vi "ReadRootPath.vi"(1 "LibBuildRootFolderName":string="ECU_Diagnose") -> (15 "Root path":path)   [LabVIEW 2020, in "DAQ.lvlib" / "DAQ_Base.lvclass"]
uses:
  DAQ_Base.lvclass
panel:
  out "匹配后偏移量":i32
  out "匹配后偏移量":i32
  out "子字符串之前":string
  out "应用程序:类别":T1(ring)
  out "原本路径":path
  # "以builds命名，并且exe直接放在builds下就不需要填这个"
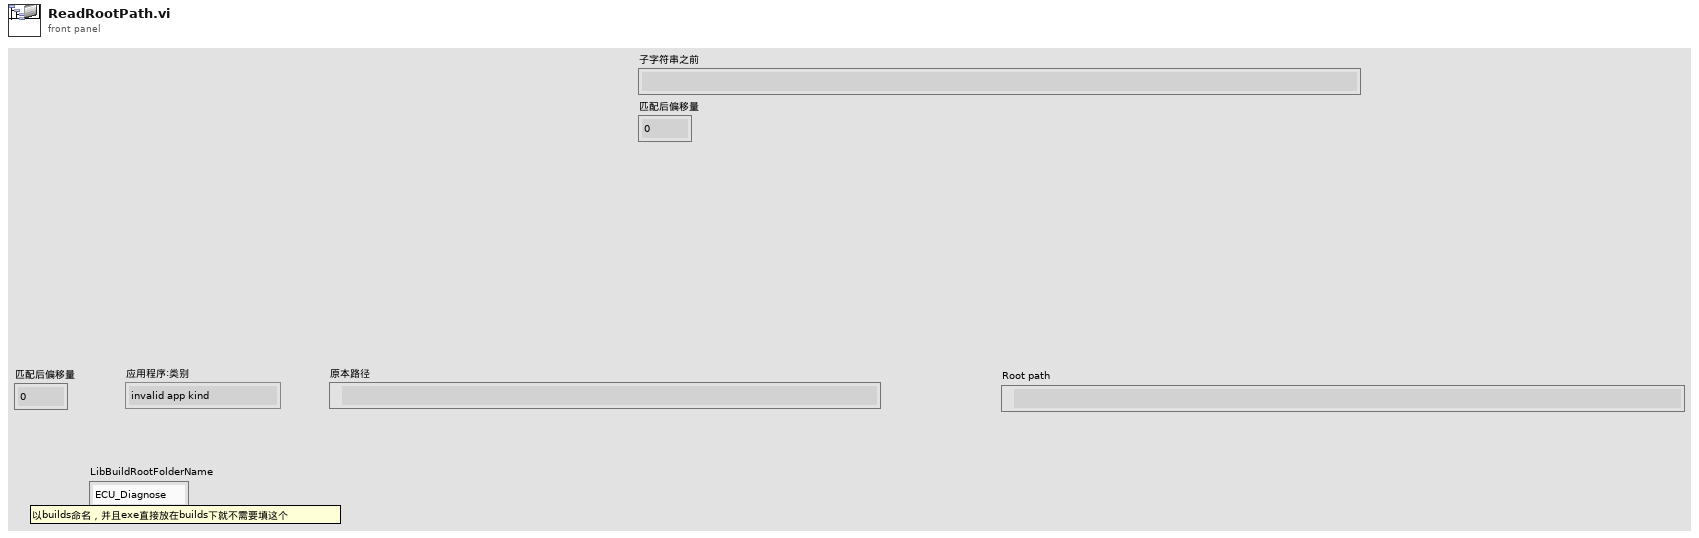
[diagram p1: front panel]
types:
  T1 = enum32{"invalid app kind", "Development System", "Run Time System", "Student Edition", "Embedded LabVIEW", "Evaluation", "Custom"}
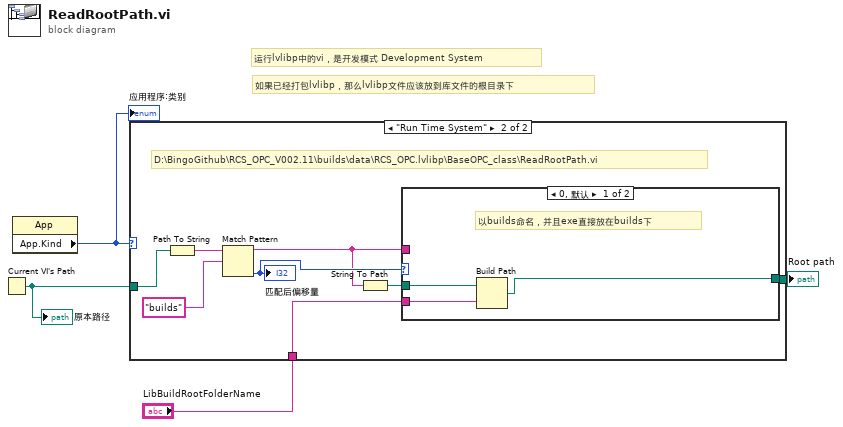
[diagram p0: block diagram]
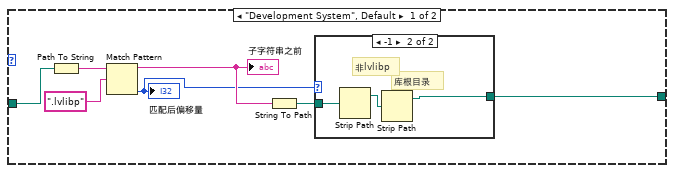
[diagram p2: hidden frame]
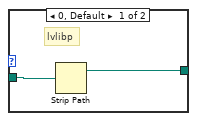
[diagram p3: hidden frame]
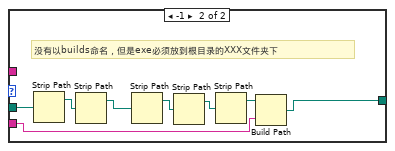
[diagram p4: hidden frame]
diagram:
  # "如果已经打包lvlibp，那么lvlibp文件应该放到库文件的根目录下"
  # "运行lvlibp中的vi，是开发模式 Development System"
  n1 = Current VI's Path() -> (path=w4:path)
  "原本路径" <- w4
  n2 = property class="App"() -> ("App.Kind"=w2:T1)  [unwired: 2 in, 2 out]
  "应用程序:类别" <- w2
  n3 = case shown="\"Run Time System\"" w2 {
    tunnel: w4 -> [w10 w20]
    tunnel: [w11 w19] -> w3
    tunnel: "LibBuildRootFolderName" -> [_ w17]
    frame "Development System", Default {
      n4 = Path To String(path=w10) -> (string=w9:string)
      n5 = Match Pattern(string=w9, regular expression=".lvlibp" ("搜索字符串")) -> (before substring=w8:string, offset past match=w6:i32)  [unwired: 1 in, 2 out]
      "子字符串之前" <- w8
      "匹配后偏移量" <- w6
      n6 = String To Path(string=w8) -> (path=w7:path)
      n7 = case shown="-1" w6 {
        tunnel: [w12 w15] -> w11
        tunnel: w7 -> [w13 w14]
        frame 0, Default {
          # "lvlibp"
          n8 = Strip Path(path=w13) -> (stripped path=w12:path)  [unwired: 1 out]
        }
        frame -1 {
          # "非lvlibp"
          # "库根目录"
          n9 = Strip Path(path=w14) -> (stripped path=w16:path)  [unwired: 1 out]
          n10 = Strip Path(path=w16) -> (stripped path=w15:path)  [unwired: 1 out]
        }
      }
    }
    frame "Run Time System" {
      # "D:\\BingoGithub\\RCS_OPC_V002.11\\builds\\data\\RCS_OPC.lvlibp\\BaseOPC_class\\ReadRootPath.vi"
      n11 = Path To String(path=w20) -> (string=w24:string)
      n12 = Match Pattern(string=w24, regular expression="builds" ("搜索字符串")) -> (before substring=w18:string, offset past match=w22:i32)  [unwired: 1 in, 2 out]
      "匹配后偏移量" <- w22
      n13 = String To Path(string=w18) -> (path=w23:path)
      n14 = case shown="0, 默认" w22 {
        tunnel: [w25 w28] -> w19
        tunnel: w23 -> [w27 w34]
        tunnel: w18 -> [_ _]
        tunnel: w17 -> [w26 w29]
        frame 0, Default {
          # "以builds命名，并且exe直接放在builds下"
          n15 = Build Path(base path=w27, name or relative path=w26) -> (appended path=w25:path)
        }
        frame -1 {
          # "没有以builds命名，但是exe必须放到根目录的XXX文件夹下"
          n16 = Strip Path(path=w34) -> (stripped path=w35:path)  [unwired: 1 out]
          n17 = Strip Path(path=w35) -> (stripped path=w32:path)  [unwired: 1 out]
          n18 = Strip Path(path=w32) -> (stripped path=w33:path)  [unwired: 1 out]
          n19 = Strip Path(path=w33) -> (stripped path=w31:path)  [unwired: 1 out]
          n20 = Strip Path(path=w31) -> (stripped path=w30:path)  [unwired: 1 out]
          n21 = Build Path(base path=w30, name or relative path=w29) -> (appended path=w28:path)
        }
      }
    }
  }
  "Root path" <- w3
